vi "Write pGames.vi"(8 "error in (no error)":errorcluster, 10 "pGames":i32, 11 "bbPlayers in":refnum<class "bbPlayers.lvclass">) -> (0 "error out":errorcluster, 3 "bbPlayers out":refnum<class "bbPlayers.lvclass">)   [LabVIEW 2020, in "ORM_Examples.lvlib" / "bbPlayers.lvclass"]
doc: "Write a new value for pGames."
uses:
  bbPlayers.lvclass
  bbPlayers.lvclass/bbPlayers.ctl
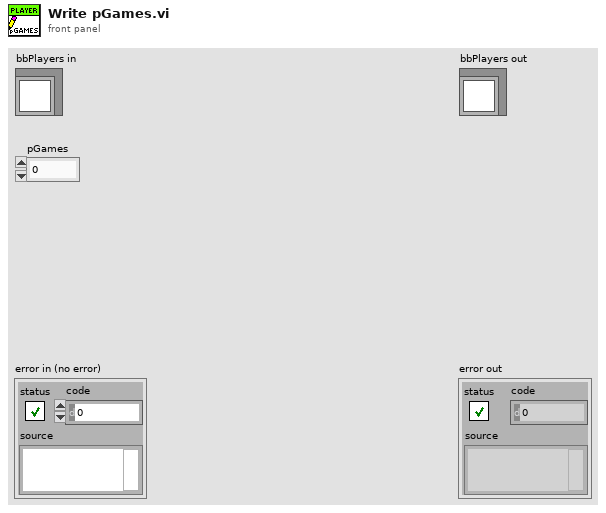
[diagram p1: front panel]
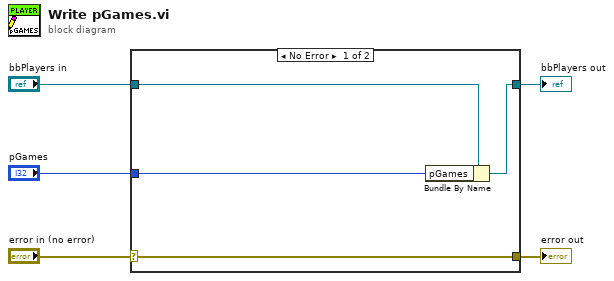
[diagram p0: block diagram]
diagram:
  n1 = case shown="No Error" "error in (no error)" {
    selector: "error in (no error)" -> [w9 w10]
    tunnel: [w9 w10] -> w4
    tunnel: [w7 w11] -> w2
    tunnel: "bbPlayers in" -> [w8 w11]
    tunnel: "pGames" -> [w6 _]
    frame No Error {
      n2 = Bundle By Name(cluster=w8, "pGames"=w6) -> (w7:refnum<class "bbPlayers.lvclass">)
    }
    frame Error {
    }
  }
  "error out" <- w4
  "bbPlayers out" <- w2
